vi "Pre Loop Init.vi"(8 "error in":errorcluster, 10 "Ref In":refnum<vi>) -> (0 "error out":errorcluster, 3 "Event Registration Refnum":refnum<event-registration>)   [LabVIEW 2018, in "Entry Console.lvlib"]
uses:
  Entry Console.lvlib
  Private Controls/Module Data Cluster.ctl
  Private Controls/Module Action.ctl
  User Events/controls/Actions.ctl
  Private Controls/Queue FG Action.ctl
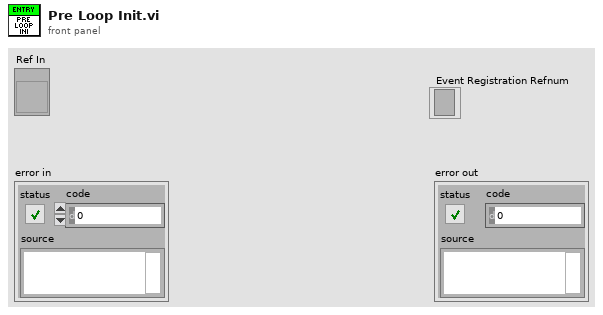
[diagram p1: front panel]
types:
  T1 = typedef "Entry Console.lvlib/Queue FG Action.ctl" = enum16{"Release", "Get", "Set"}
  T2 = typedef "Actions.ctl" = enum16{"Get", "Create", "Destroy"}
  T3 = typedef "Entry Console.lvlib/Module Data Cluster.ctl" = cluster{"Variant":variant, "action":T4}
  T4 = typedef "Entry Console.lvlib/Module Action.ctl" = enum16{"error", "exit", "Start Wash", "init", "Enable Wash Buttons"}
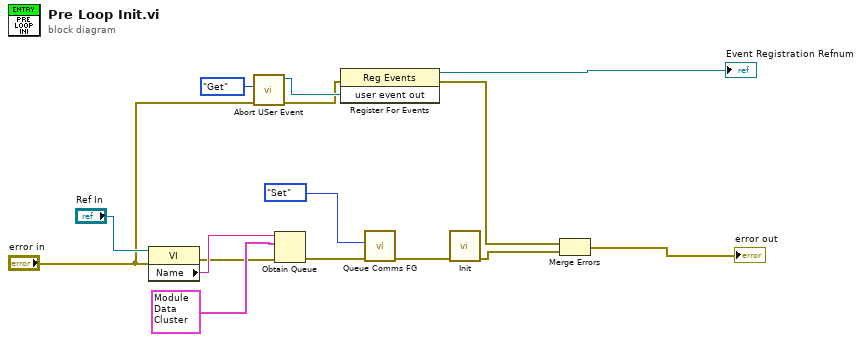
[diagram p0: block diagram]
diagram:
  n1 = property class="VI"(reference="Ref In", error in="error in") -> (error out=w8:errorcluster, "Name"=w14:string)  [unwired: 1 out]
  n2 = call "Abort USer Event.vi"("error in"="error in", "Enum"=Actions."Get") -> ("error out"=w2:errorcluster, "user event out"=w5:refnum<user-event>)  [unwired: 8 in]
  n3 = Obtain Queue(name (unnamed)=w14, element data type=T3 {"Variant"=variant, "action"=enum."init"} ("Module Data Cluster"), error in (no error)=w8) -> (error out=w12:errorcluster)  [unwired: 2 in, 2 out]
  n4 = register-events(error in=w2, w5) -> (reference out=→"Event Registration Refnum":refnum<event-registration>, error out=w4:errorcluster)  [unwired: 1 in]
  n5 = call "Queue Comms FG.vi"("error in"=w12, "Action"=Queue_FG_Action."Set") -> ("error out"=w11:errorcluster)  [unwired: 8 in, 1 out]
  n6 = call "Init.vi"("error in"=w11) -> ("error out"=w10:errorcluster)  [unwired: 10 in]
  n7 = Merge Errors(w4, w10) -> (→"error out":errorcluster)
